vi "Tele_Solenoid.vi"(8 "Button B":bool, 9 "Button A":bool, 10 "Solenoid B":string="Shooter High Out", 11 "Solenoid A":string="Shooter High In") -> ()   [LabVIEW 2013]
uses:
  <vilib>/Rock Robotics/WPI/Relay/WPI_RelayValue.ctl
  <vilib>/Rock Robotics/WPI/Solenoid/WPI_SolenoidSetEnum.vi
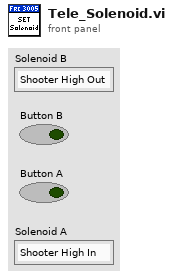
[diagram p1: front panel]
types:
  T1 = typedef "WPI_RelayValue.ctl" = enum16{"Off", "On", "Forward", "Reverse"}
  T2 = typedef "WPI_SolenoidDevRef.ctl" = cluster{"DevStatus":errorcluster, "Solenoid Module":T3, "Forward Solenoid Channel":T4, "Reverse Solenoid Channel":T4}
  T3 = typedef "FPGA_TypedefSolenoidModule.ctl" = enum16{"Solenoid Module 1", "Solenoid Module 2"}
  T4 = typedef "WPI_SolenoidChannel.ctl" = enum8{"Solenoid 1", "Solenoid 2", "Solenoid 3", "Solenoid 4", "Solenoid 5", "Solenoid 6", "Solenoid 7", "Solenoid 8", "Invalid"}
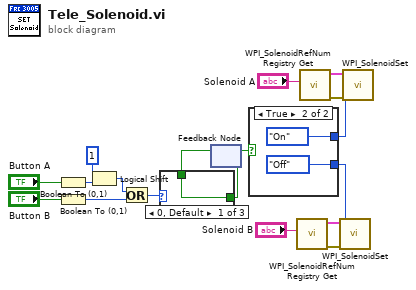
[diagram p0: block diagram]
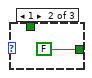
[diagram p2: hidden frame]
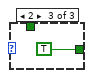
[diagram p3: hidden frame]
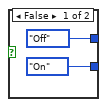
[diagram p4: hidden frame]
diagram:
  n1 = Boolean To (0,1)(Boolean="Button A") -> (0, 1=w10:i16)
  n2 = Boolean To (0,1)(Boolean="Button B") -> (0, 1=w13:i16)
  n3 = Logical Shift(y=i16 1, x=w10) -> (x << y=w12:i16)
  n4 = Or(x=w12, y=w13) -> (x .or. y?=w7:i16)
  n5 = feedback #1() -> (w14:bool)  [unwired: 1 in]
  n6 = case shown="0, Default" w7 {
    tunnel: [w18 FALSE TRUE] -> w15
    tunnel: w14 -> [w18 _ _]
    frame 0, Default {
    }
    frame 1 {
    }
    frame 2 {
    }
  }
  n7 = feedback-in #1(w15) -> ()
  n8 = case shown="True" w15 {
    tunnel: [WPI_RelayValue."Off" ("RelayValue") WPI_RelayValue."On" ("RelayValue")] -> w17
    tunnel: [WPI_RelayValue."On" ("RelayValue") WPI_RelayValue."Off" ("RelayValue")] -> w16
    frame False {
    }
    frame True {
    }
  }
  n9 = call <vilib>:"WPI_SolenoidRefNum Registry Get.vi"("refnum name"="Solenoid B") -> ("error out"=w2:errorcluster, "SolenoidDevRef"=w3:T2)  [unwired: 9 in]
  n10 = call <vilib>:"WPI_SolenoidRefNum Registry Get.vi"("refnum name"="Solenoid A") -> ("error out"=w5:errorcluster, "SolenoidDevRef"=w4:T2)  [unwired: 9 in]
  n11 = call-poly <vilib>:"WPI_SolenoidSet.vi"("error in (no error)"=w2, "Value"=w16, "SolenoidDevRef"=w3) -> ()  [unwired: 7 in, 2 out]
  n12 = call-poly <vilib>:"WPI_SolenoidSet.vi"("error in (no error)"=w5, "Value"=w17, "SolenoidDevRef"=w4) -> ()  [unwired: 7 in, 2 out]
